vi "TestStandApplicationManager.vi"(7 "action":T1, 8 "error in":errorcluster) -> (0 "error out":errorcluster, 2 "TestStand UI Application Manager":refnum<k7>)   [LabVIEW 2019, in "Tools.lvlib"]
uses:
  Tools.lvlib
  TestStandApplicationManager.Action.ctl
panel:
  in  "TestStand UI Application Manager":refnum<k7>(container)
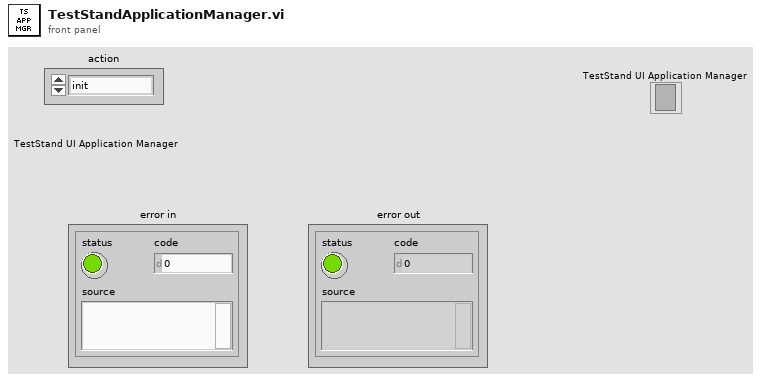
[diagram p1: front panel]
types:
  T1 = typedef "Tools.lvlib/TestStandApplicationManager.Action.ctl" = enum16{"init", "get", "start", "release", "close all sequence files", "close all executions", "shutdown"}
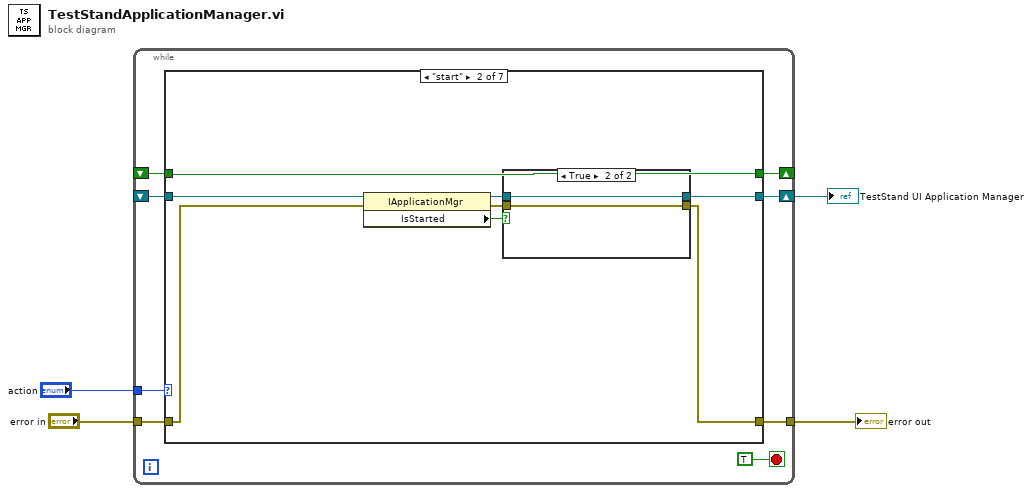
[diagram p0: block diagram]
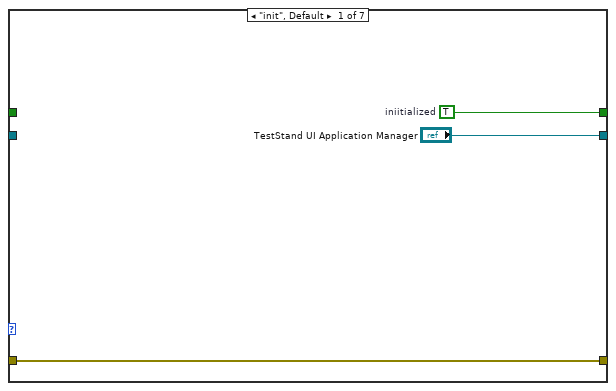
[diagram p2: hidden frame]
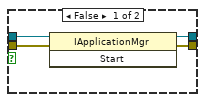
[diagram p3: hidden frame]
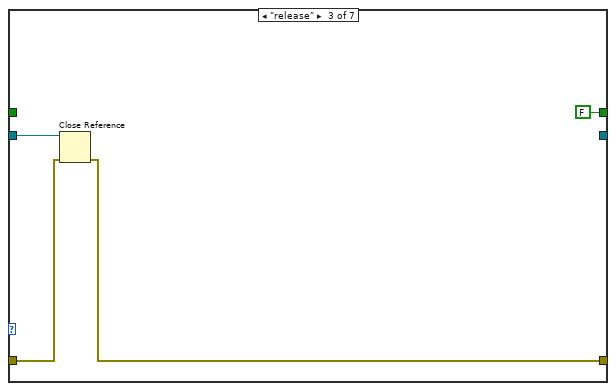
[diagram p4: hidden frame]
diagram:
  n1 = while {
    shift-right: [w10] -> w3
    shift-left: _ -> [w7]
    tunnel: "action" -> [w11]
    shift-right: [w9] -> _
    shift-left: _ -> [w8]
    tunnel: "error in" -> [w6]
    tunnel: [w5] -> w1
    stop <- TRUE stop-if-true
    n2 = case shown="\"start\"" w11 {
      tunnel: ["TestStand UI Application Manager" w19 _ w35 w38 w41 w44] -> w10
      tunnel: [w14 w18 FALSE ("iniitialized") w36 w39 w42 w45] -> w9
      tunnel: w8 -> [_ w18 _ w36 w39 w42 w45]
      tunnel: w7 -> [_ w17 w33 w35 w38 w41 w44]
      tunnel: w6 -> [w13 w16 w32 w34 w37 w40 w43]
      tunnel: [w13 w20 w31 w34 w37 w40 w43] -> w5
      frame "init", Default {
        w14 = TRUE  # iniitialized
      }
      frame "start" {
        n3 = property class="IApplicationMgr"(reference=w17, error in=w16) -> (reference out=w23:refnum<k7>, error out=w22:errorcluster, "IsStarted"=w21:bool)
        n4 = case shown="True" w21 {
          tunnel: [w27 w28] -> w19
          tunnel: [w26 w29] -> w20
          tunnel: w22 -> [w25 w29]
          tunnel: w23 -> [w24 w28]
          frame False {
            n5 = invoke class="IApplicationMgr" method="Start"(reference=w24, error in=w25) -> (reference out=w27:refnum<k7>, error out=w26:errorcluster)  [unwired: 1 in, 1 out]
          }
          frame True {
          }
        }
      }
      frame "release" {
        n6 = Close Reference(reference=w33, error in (no error)=w32) -> (error out=w31:errorcluster)
      }
      frame "close all sequence files" {
      }
      frame "close all executions" {
      }
      frame "shutdown" {
      }
      frame "get" {
      }
    }
  }
  "TestStand UI Application Manager" <- w3
  "error out" <- w1
